vi "test_AllowedCharsInName_CheckPluginNameIsValid_NameValid.vi"() -> (6 "pass":bool, 8 "result":string, 15 "error out":errorcluster)   [LabVIEW 2021]
uses:
  <vilib>/ErrorRing/Error Ring.xnode
  Generator/_Editor/Generator Helpers.lvlib
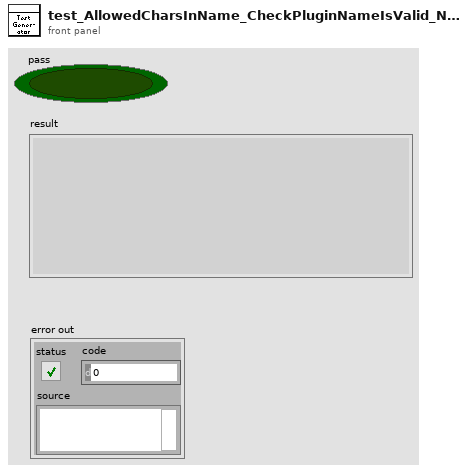
[diagram p1: front panel]
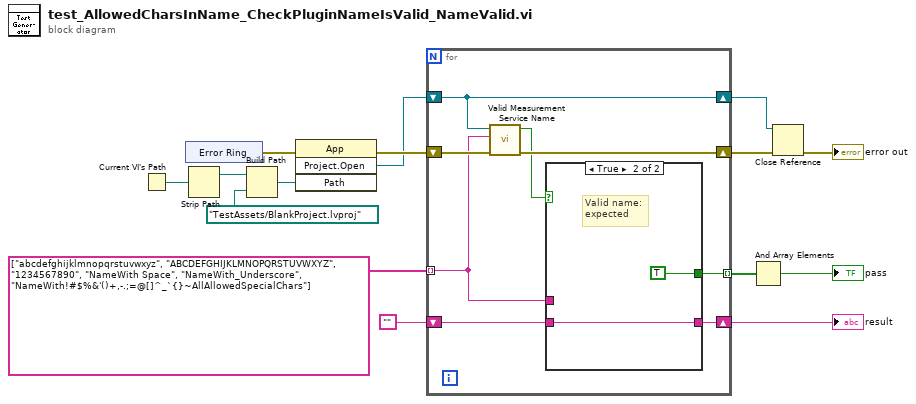
[diagram p0: block diagram]
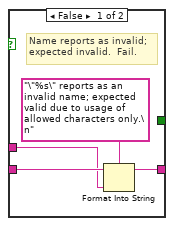
[diagram p2: hidden frame]
diagram:
  n1 = Current VI's Path() -> (path=w15:path)
  n2 = xnode "Error Ring"() -> ("error out"=w12:errorcluster)
  n3 = Strip Path(path=w15) -> (stripped path=w14:path)  [unwired: 1 out]
  n4 = Build Path(base path=w14, name or relative path=path "TestAssets/BlankProject.lvproj" ("path")) -> (appended path=w11:path)
  n5 = invoke class="App" method="Project.Open"(error in=w12, "Path"=w11) -> (error out=w3:errorcluster, "Project:Open"=w2:refnum<vi>)  [unwired: 2 in, 2 out]
  n6 = for {
    shift-right: [w22] -> w10
    shift-left: w3 -> [w23]
    tunnel: string[] ["abcdefghijklmnopqrstuvwxyz", "ABCDEFGHIJKLMNOPQRSTUVWXYZ", "1234567890", "NameWith Space", "NameWith_Underscore", "NameWith!#$%&'()+,-.;=@[]^_`{}~AllAllowedSpecialChars"] -> [w16] mode=indexing
    shift-right: [w21] -> w8
    shift-left: w2 -> [w21]
    shift-right: [w18] -> w6
    shift-left: "" -> [w19]
    tunnel: [w17] -> w5 mode=indexing
    n7 = call "Valid Measurement Service Name.vi"("error in"=w23, "requested plugin name"=w16, "project ref"=w21) -> ("error out"=w22:errorcluster, "valid name?"=w20:bool)  [unwired: 7 in]
    n8 = case shown="True" w20 {
      tunnel: w19 -> [w27 w29]
      tunnel: [w26 w29] -> w18
      tunnel: [_ TRUE] -> w17
      tunnel: w16 -> [w25 _]
      frame False {
        # "Name reports as invalid;\nexpected invalid.  Fail."
        n9 = Format Into String(format string="\"%s\" reports as an invalid name; expected valid due to usage of allowed characters only.\n", initial string=w27, w25) -> (resulting string=w26:string)  [unwired: 1 in, 1 out]
      }
      frame True {
        # "Valid name:\nexpected"
      }
    }
  }
  "result" <- w6
  n10 = And Array Elements(Boolean array=w5) -> (logical AND=→"pass":bool)
  n11 = Close Reference(reference=w8, error in (no error)=w10) -> (error out=→"error out":errorcluster)
